vi "KG set pump_a.vi"(8 "Fehler (Eingang, kein Fehler)":errorcluster, 9 "A":dbl, 10 "pump":u32, 11 "VISA-Ressourcenname":refnum<visa-resource-name>) -> (0 "Fehler (Ausgang)":errorcluster, 2 "Kommando gesendet":string, 3 "VISA-Ressourcenname (Ausgang)":refnum<visa-resource-name>)   [LabVIEW 2020, in "Linearisierung v2.lvlib" / "Gasteiler.lvlib" / "HovaCAL_Interface.lvlib" / "KGN.lvlib" / "set.lvlib"]
uses:
  set.lvlib
  KGN.lvlib
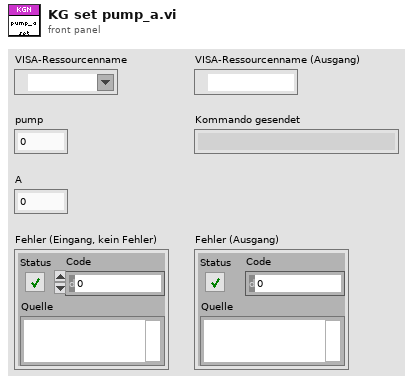
[diagram p1: front panel]
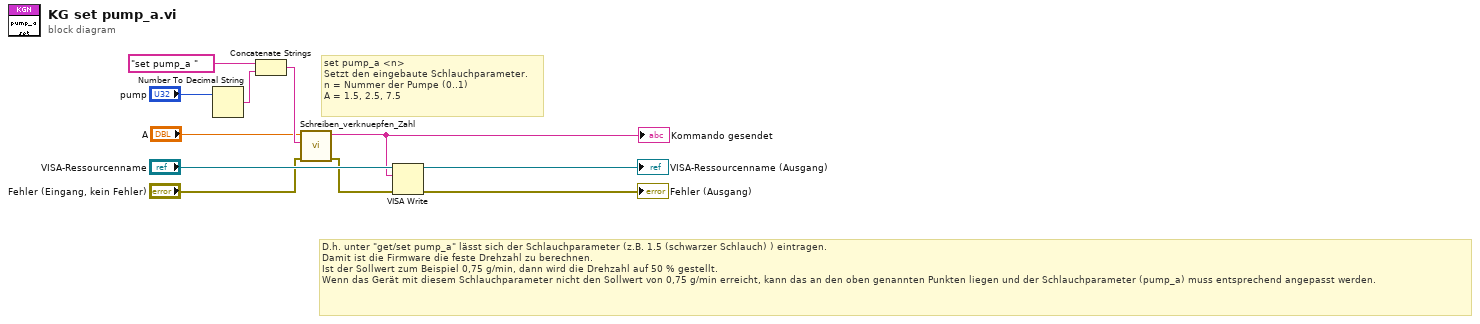
[diagram p0: block diagram]
diagram:
  # "D.h. unter \"get/set pump_a\" lässt sich der Schlauchparameter (z.B. 1.5 (schwarzer Schlauch) ) eintragen. \nDamit ist die Firmware die feste Drehzahl zu berechnen.\nIst der Sollwert zum Beispiel 0,75 g/min, dann wird die Drehzahl auf 50 % gestellt.\nWenn das Gerät mit diesem Schlauchparameter nicht den Sollwert von 0,75 g/min erreicht, kann das an den oben genannten Punkten liegen und der Schlauchparameter (pump_a) muss entsprechend angepasst werden."
  # "set pump_a <n>\nSetzt den eingebaute Schlauchparameter.\nn = Nummer der Pumpe (0..1)\nA = 1.5, 2.5, 7.5"
  n1 = Number To Decimal String(number="pump") -> (decimal integer string=w2:string)  [unwired: 1 in]
  n2 = Concatenate Strings("set pump_a " ("Schreibpuffer"), w2) -> (w3:string)
  n3 = call "Schreiben_verknuepfen_Zahl.vi"("error in (no error)"="Fehler (Eingang, kein Fehler)", "Order"=w3, "Zahl"="A") -> ("error out"=w6:errorcluster, "Verknüpfter String"=w5:string)  [unwired: 7 in]
  "Kommando gesendet" <- w5
  n4 = VISA Write(VISA resource name="VISA-Ressourcenname", write buffer=w5, error in (no error)=w6) -> (VISA resource name out=→"VISA-Ressourcenname (Ausgang)":refnum<visa-resource-name>, error out=→"Fehler (Ausgang)":errorcluster)  [unwired: 1 out]
